vi "Ctor.vi"(8 "error in (no error)":errorcluster, 11 "ControlBindingPanel in":refnum<class "ControlBindingPanel.lvclass">) -> (0 "error out":errorcluster, 3 "ControlBindingPanel out":refnum<class "ControlBindingPanel.lvclass">)   [LabVIEW 2020, in "VolatusGUIEditor.lvlib" / "ControlBindingPanel.lvclass"]
uses:
  ControlBindingPanel.lvclass
  ControlBindingPanel.lvclass/ControlBindingPanel.ctl
  lv-oopanel/OOPanel/Panel/Panel.lvclass
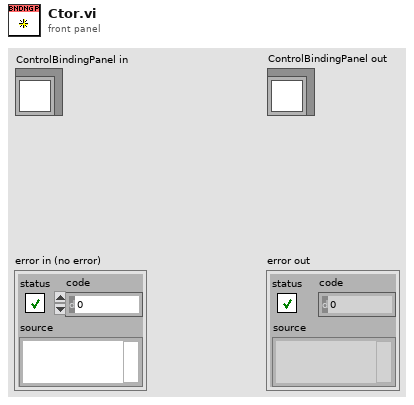
[diagram p1: front panel]
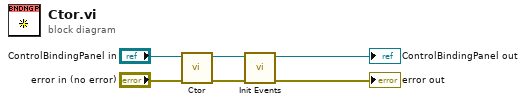
[diagram p0: block diagram]
diagram:
  n1 = call-parent "Ctor.vi"("error in (no error)"="error in (no error)", "Panel in"="ControlBindingPanel in") -> ("error out"=w3:errorcluster, "Panel out"=w1:refnum<class "ControlBindingPanel.lvclass">)  [unwired: 8 in]
  n2 = call "Init Events.vi"("error in (no error)"=w3, "ControlBindingPanel in"=w1) -> ("error out"=→"error out":errorcluster, "ControlBindingPanel out"=→"ControlBindingPanel out":refnum<class "ControlBindingPanel.lvclass">)  [unwired: 8 in]
